vi "Close Stream VI.vi"(8 "error in (no error)":errorcluster, 11 "Channel in":refnum<class "Channel.lvclass">) -> (0 "error out":errorcluster, 3 "Channel out":refnum<class "Channel.lvclass">)   [LabVIEW 2018, in "Channel.lvclass"]
uses:
  Channel.lvclass
  Channel.lvclass/Channel.ctl
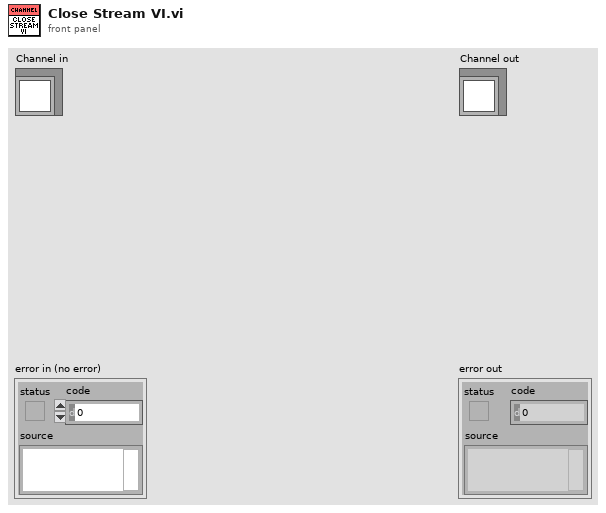
[diagram p1: front panel]
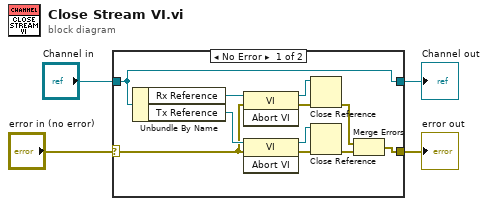
[diagram p0: block diagram]
diagram:
  n1 = case shown="No Error" "error in (no error)" {
    selector: "error in (no error)" -> [w10 w17]
    tunnel: [w9 w17] -> w2
    tunnel: [w15 w16] -> w1
    tunnel: "Channel in" -> [w15 w16]
    frame No Error {
      n2 = Unbundle By Name(w15) -> ("Rx Reference"=w13:refnum<vi>, "Tx Reference"=w14:refnum<vi>)
      n3 = invoke class="VI" method="Abort VI"(reference=w13, error in=w10) -> (reference out=w12:refnum<vi>, error out=w8:errorcluster)  [unwired: 1 in, 1 out]
      n4 = invoke class="VI" method="Abort VI"(reference=w14, error in=w10) -> (reference out=w11:refnum<vi>, error out=w6:errorcluster)  [unwired: 1 in, 1 out]
      n5 = Close Reference(reference=w12, error in (no error)=w8) -> (error out=w7:errorcluster)
      n6 = Close Reference(reference=w11, error in (no error)=w6) -> (error out=w5:errorcluster)
      n7 = Merge Errors(w7, w5) -> (w9:errorcluster)
    }
    frame Error {
    }
  }
  "error out" <- w2
  "Channel out" <- w1
